vi "Acquisition_c.vi"() -> (4 "Acquired_Data":dbl(graph))   [LabVIEW 2021]
doc: "This VI acquire data that were generated be the Generator VI.\nTransfer of thet data happens under Queue LV2."
uses:
  Type_Def/Operation_Queue.ctl
panel:
  out "Error_Out":errorcluster
  in  "Error_In":errorcluster
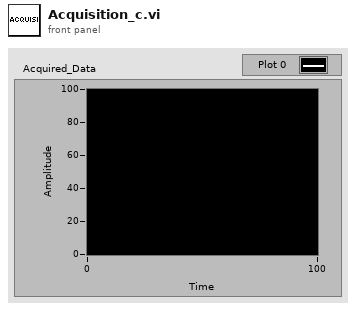
[diagram p1: front panel]
types:
  T1 = typedef "Operation_Queue.ctl" = enum16{"Initialize", "Enqueue", "Dequeue", "Sum"}
  T2 = enum16{"Left Button", "Center Button", "Right Button", "Window Close"}
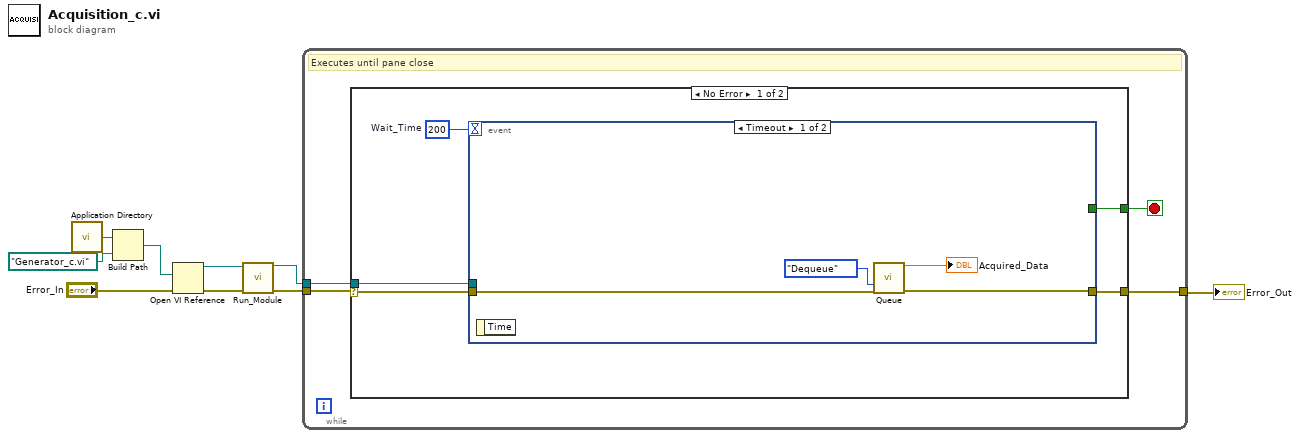
[diagram p0: block diagram]
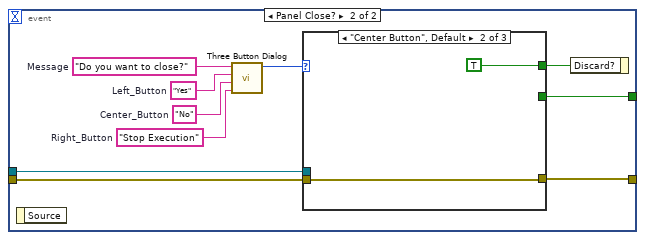
[diagram p2: hidden frame]
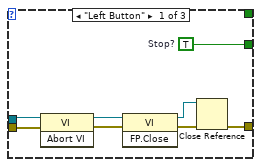
[diagram p3: hidden frame]
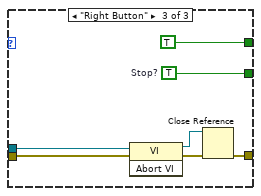
[diagram p4: hidden frame]
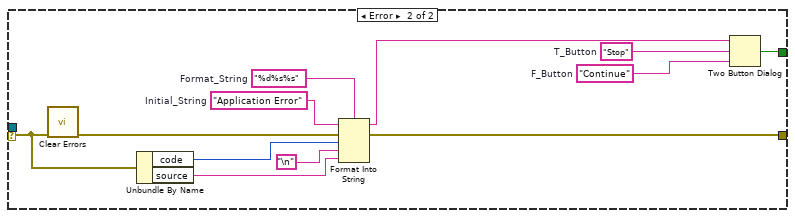
[diagram p5: hidden frame]
diagram:
  n1 = call <vilib>:"Application Directory.vi"() -> ("Application Directory"=w7:path)
  n2 = Build Path(base path=w7, name or relative path=path "Generator_c.vi") -> (appended path=w8:path)
  n3 = Open VI Reference(vi path=w8, error in (no error)="Error_In") -> (vi reference=w2:refnum<vi>, error out=w4:errorcluster)  [unwired: 4 in]
  n4 = call "Run_Module.vi"("VI_In"=w2, "Error_In"=w4) -> ("VI_Out"=w3:refnum<vi>, "Error_Out"=w1:errorcluster)  [unwired: 12 in]
  n5 = while {
    tunnel: w1 -> [w12]
    tunnel: [w11] -> w5
    tunnel: w3 -> [w10]
    stop <- w13 stop-if-true
    # "Executes until pane close"
    n6 = case shown="No Error" w12 {
      selector: w12 -> [w16 w55]
      tunnel: [w17 w50] -> w13
      tunnel: [w15 w53] -> w11
      tunnel: w10 -> [w14 _]
      frame No Error {
        w18 = 200  # Wait_Time
        n7 = event shown="[0] Timeout" {
          selector: _ -> [_ _]
          dyn-events: _ -> [_ _]
          timeout: w18 -> [_ _]
          tunnel: [_ w26] -> w17
          tunnel: w16 -> [w22 w24]
          tunnel: [w21 w25] -> w15
          tunnel: w14 -> [_ w23]
          event Timeout {
            n8 = event-data() -> ()  [unwired: 1 in, 1 out]
            n9 = call "Queue.vi"("Operation"=Operation_Queue."Dequeue" ("Operation_Queue"), "Error_In"=w22) -> ("Element_Out"=→"Acquired_Data":dbl, "Error_Out"=w21:errorcluster)  [unwired: 9 in, 3 out]
          }
          event Panel Close? {
            w29 = "Stop Execution"  # Right_Button
            w30 = "No"  # Center_Button
            w31 = "Yes"  # Left_Button
            w32 = "Do you want to close?"  # Message
            n10 = event-data() -> ()  [unwired: 1 in, 1 out]
            n11 = call <vilib>:"Three Button Dialog.vi"("Right Button Text (\"Cancel\")"=w29, "Center Button Text (\"No\")"=w30, "Left Button Text (\"Yes\")"=w31, "message"=w32) -> ("Which Button?"=w28:T2)  [unwired: 7 in]
            n12 = case shown="\"Center Button\", Default" w28 {
              tunnel: [_ TRUE ("Discard?") TRUE ("Discard?")] -> w27
              tunnel: [w40 _ w49] -> w26
              tunnel: [w37 w41 w45] -> w25
              tunnel: w24 -> [w34 w41 w44]
              tunnel: w23 -> [w35 _ w43]
              frame "Left Button" {
                w40 = TRUE  # Stop?
                n13 = invoke class="VI" method="Abort VI"(reference=w35, error in=w34) -> (reference out=w36:refnum<vi>, error out=w33:errorcluster)  [unwired: 1 in, 1 out]
                n14 = invoke class="VI" method="FP.Close"(reference=w36, error in=w33) -> (reference out=w39:refnum<vi>, error out=w38:errorcluster)  [unwired: 1 in, 1 out]
                n15 = Close Reference(reference=w39, error in (no error)=w38) -> (error out=w37:errorcluster)
              }
              frame "Center Button", Default {
              }
              frame "Right Button" {
                w49 = TRUE  # Stop?
                n16 = invoke class="VI" method="Abort VI"(reference=w43, error in=w44) -> (reference out=w47:refnum<vi>, error out=w46:errorcluster)  [unwired: 1 in, 1 out]
                n17 = Close Reference(reference=w47, error in (no error)=w46) -> (error out=w45:errorcluster)
              }
            }
            n18 = event-data ("Event Filter Node")("Discard?"=w27) -> ()  [unwired: 1 in, 1 out]
          }
        }
      }
      frame Error {
        w57 = "%d%s%s"  # Format_String
        w58 = "Application Error"  # Initial_String
        w59 = "Stop"  # T_Button
        w60 = "Continue"  # F_Button
        n19 = call <vilib>:"Clear Errors.vi"("error in (no error)"=w55) -> ("error out"=w54:errorcluster)  [unwired: 5 in, 1 out]
        n20 = Unbundle By Name(w55) -> ("code"=w52:i32, "source"=w51:string)
        n21 = Format Into String(format string=w57, initial string=w58, error in=w54, w52, "\n", w51) -> (resulting string=w61:string, error out=w53:errorcluster)
        n22 = Two Button Dialog(message=w61, 1:w60, 2:w59) -> (T button?=w50:bool)
      }
    }
  }
  "Error_Out" <- w5
